vi "Is Call Cancelled Global.vi"() -> ()   [LabVIEW 2019]
panel:
  out "Is Call Cancelled?":bool
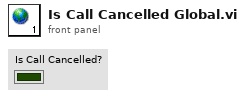
[diagram p1: front panel]
diagram:
